vi "Set Message2.vi"   [LabVIEW 2015]
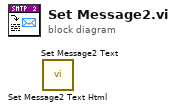
[diagram p0: block diagram]
diagram:
  n1 = call "Set Message2 Text Html.vi"() -> ()  [unwired: 14 in, 2 out]
  n2 = call "Set Message2 Text.vi"() -> ()  [unwired: 14 in, 2 out]
